vi "Help Center.vi"() -> ()   [LabVIEW 2014]
uses:
  <vilib>/Platform/TimedLoop/XDataNode/timing_clust.ctl
  <vilib>/Platform/TimedLoop/XDataNode/nitl_modes.ctl
  <vilib>/Platform/TimedLoop/XDataNode/wakeup.ctl
  <vilib>/Platform/TimedLoop/XDataNode/XDataNode.xnode
  <vilib>/Platform/TimedLoop/XDataNode/XDNodeRunTimeDep.lvlib
panel:
  in  "Close Button":bool
  in  "Help Tree":string(tree)
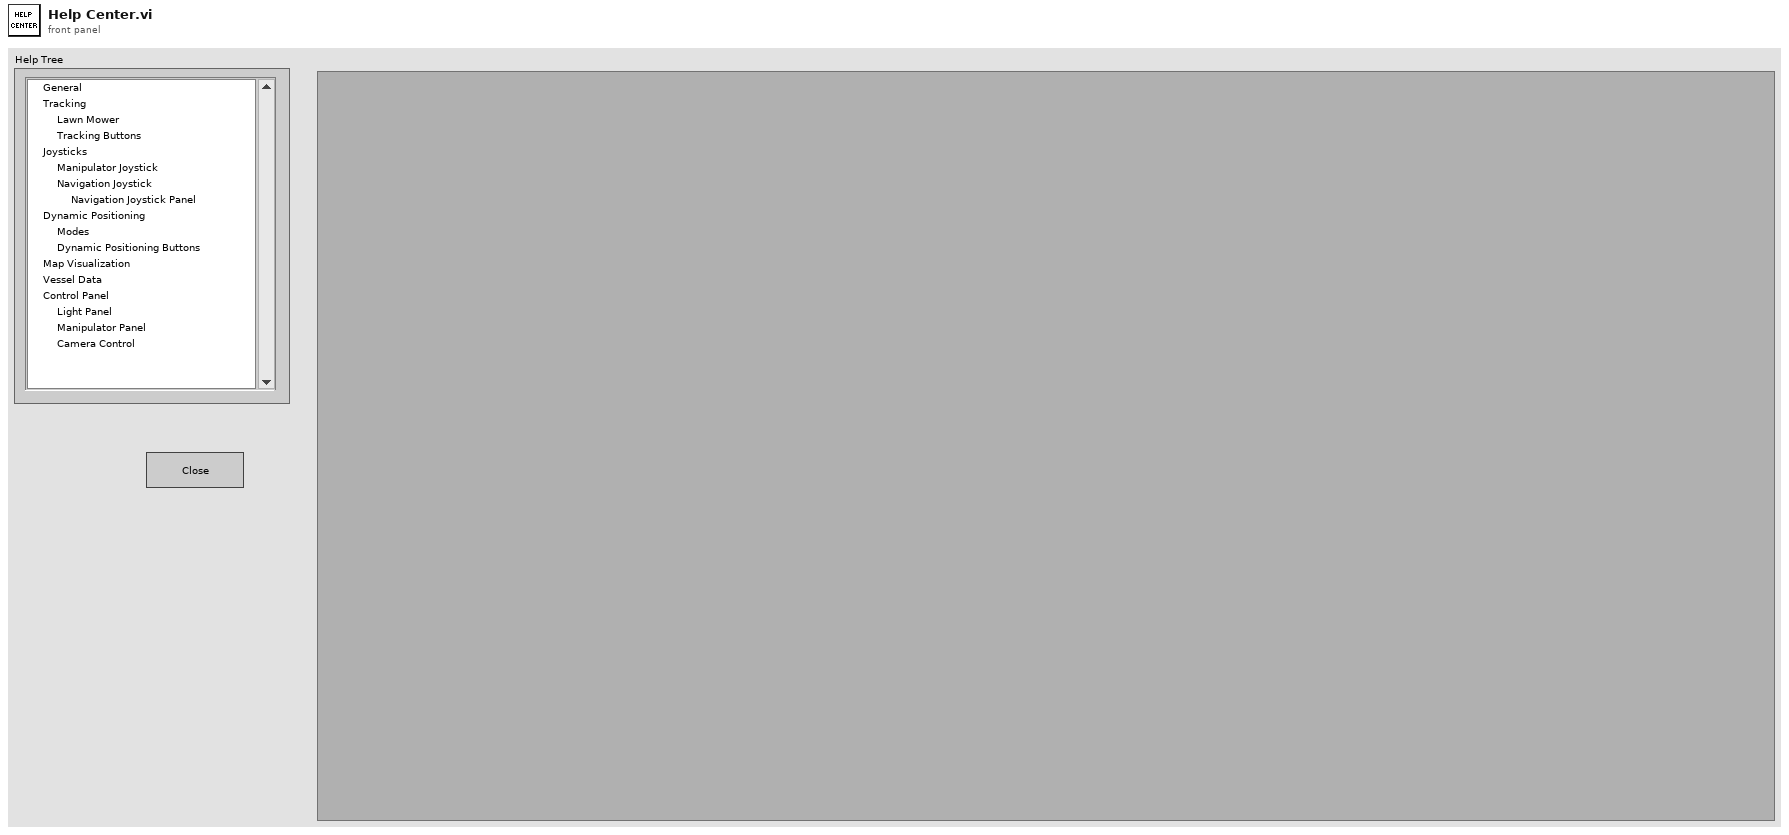
[diagram p1: front panel]
types:
  T1 = typedef "XDNodeRunTimeDep.lvlib/timing_clust.ctl" = cluster{"Expected End [f-1]":u64, "Actual End [f-1]":u64, "Finished Late? [f-1]":bool, "Expected End [i-1]":u64, "Actual End [i-1]":u64, "Finished Late? [i-1]":bool, "Expected Start [i]":u64, "Actual Start [i]":u64, "Expected Start [f]":u64, "Actual Start [f]":u64, "Source Name":string, "Structure Name":string, "Period":i64, "Deadline":i64, "Offset":i64, "Start":i64, "Priority":i32, "Timeout":i32, "Mode":T2, "Wakeup Reason":T3, "Error":errorcluster, "Source Type":string, "Secondary Source Type":string, "Global End Time":u64, "Global Start Time":u64, "Frame Duration":u64, "Iteration Duration":u64, "Assigned CPU":i32, "I/O Scan Engine Mode":u32}
  T2 = typedef "XDNodeRunTimeDep.lvlib/nitl_modes.ctl" = enum32{"No Change", "Process missed periods, maintain original phase", "Discard missed periods, maintain original phase", "Process missed periods, ignore original phase", "Discard missed periods, ignore original phase"}
  T3 = typedef "XDNodeRunTimeDep.lvlib/wakeup.ctl" = enum32{"Normal", "Aborted", "Asynchronous wakeup", "Timing source error", "Timed loop error", "Timeout"}
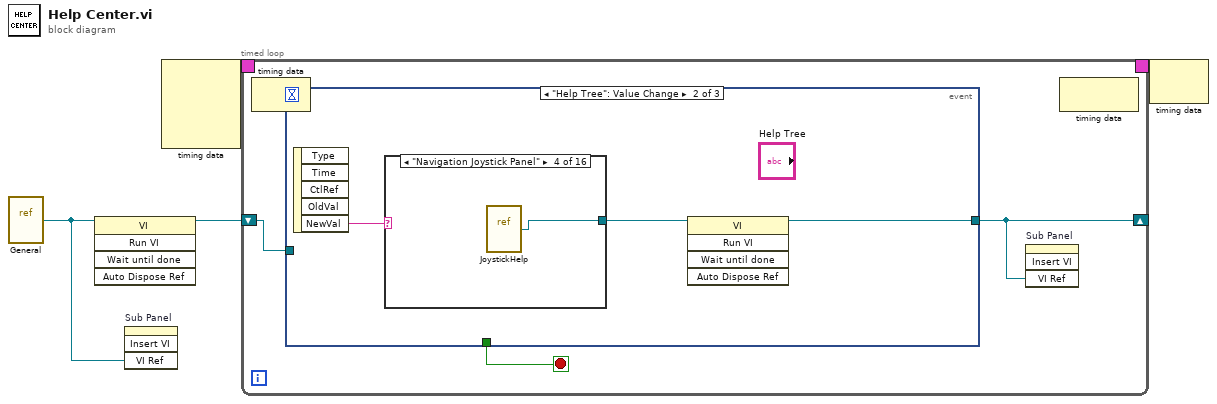
[diagram p0: block diagram]
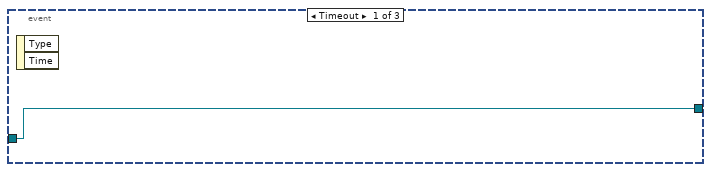
[diagram p2: hidden frame]
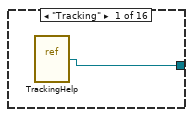
[diagram p3: hidden frame]
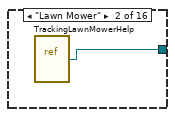
[diagram p4: hidden frame]
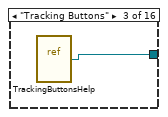
[diagram p5: hidden frame]
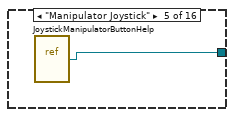
[diagram p6: hidden frame]
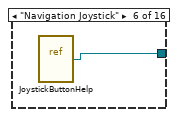
[diagram p7: hidden frame]
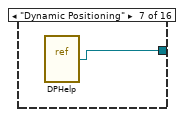
[diagram p8: hidden frame]
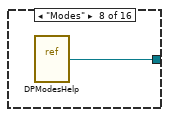
[diagram p9: hidden frame]
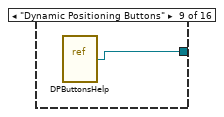
[diagram p10: hidden frame]
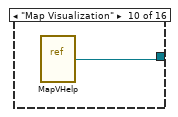
[diagram p11: hidden frame]
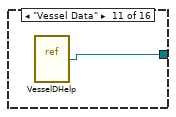
[diagram p12: hidden frame]
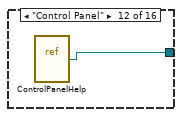
[diagram p13: hidden frame]
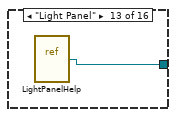
[diagram p14: hidden frame]
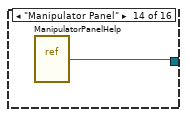
[diagram p15: hidden frame]
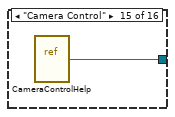
[diagram p16: hidden frame]
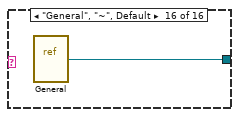
[diagram p17: hidden frame]
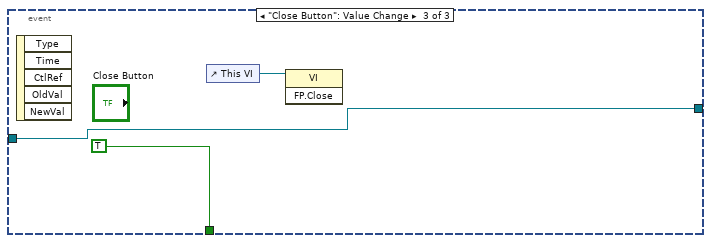
[diagram p18: hidden frame]
diagram:
  n1 = vi-ref "General.vi"() -> (w3:refnum<vi>)
  n2 = invoke class="VI" method="Run VI"(reference=w3) -> (reference out=w4:refnum<vi>)  [unwired: 4 in, 4 out]
  n3 = invoke on="Sub Panel" class="SubPnl" method="Insert VI"("VI Ref"=w3) -> ()  [unwired: 3 in, 4 out]
  n4 = node-c288() -> (w2:T1)  [unwired: 4 in]
  n5 = timed-loop {
    shift-right: [w6] -> _
    shift-left: w4 -> [w5]
    timing: w2 -> [_]
    timing-out: [_] -> w1
    stop <- w7 stop-if-true
    n6 = node-c288() -> ()  [unwired: 1 in, 1 out]
    n7 = event shown="[1] \"Help Tree\": Value Change" {
      selector: _ -> [_ _ _]
      dyn-events: _ -> [_ _ _]
      timeout: _ -> [_ _ _]
      tunnel: [_ _ TRUE] -> w7
      tunnel: [w10 w11 w30] -> w6
      tunnel: w5 -> [w10 _ w30]
      event Timeout {
        n8 = event-data() -> ()  [unwired: 1 in, 2 out]
      }
      event "Help Tree": Value Change {
        n9 = event-data() -> ("NewVal"=w13:string)  [unwired: 1 in, 4 out]
        n10 = case shown="\"Navigation Joystick Panel\"" w13 {
          tunnel: [w14 w15 w16 w17 w18 w19 w20 w21 w22 w23 w24 w25 w26 w27 w28 w29] -> w12
          frame "Tracking" {
            n11 = vi-ref "TrackingHelp.vi"() -> (w14:refnum<vi>)
          }
          frame "Lawn Mower" {
            n12 = vi-ref "TrackingLawnMowerHelp.vi"() -> (w15:refnum<vi>)
          }
          frame "Tracking Buttons" {
            n13 = vi-ref "TrackingButtonsHelp.vi"() -> (w16:refnum<vi>)
          }
          frame "Navigation Joystick Panel" {
            n14 = vi-ref "JoystickHelp.vi"() -> (w17:refnum<vi>)
          }
          frame "Manipulator Joystick" {
            n15 = vi-ref "JoystickManipulatorButtonHelp.vi"() -> (w18:refnum<vi>)
          }
          frame "Navigation Joystick" {
            n16 = vi-ref "JoystickButtonHelp.vi"() -> (w19:refnum<vi>)
          }
          frame "Dynamic Positioning" {
            n17 = vi-ref "DPHelp.vi"() -> (w20:refnum<vi>)
          }
          frame "Modes" {
            n18 = vi-ref "DPModesHelp.vi"() -> (w21:refnum<vi>)
          }
          frame "Dynamic Positioning Buttons" {
            n19 = vi-ref "DPButtonsHelp.vi"() -> (w22:refnum<vi>)
          }
          frame "Map Visualization" {
            n20 = vi-ref "MapVHelp.vi"() -> (w23:refnum<vi>)
          }
          frame "Vessel Data" {
            n21 = vi-ref "VesselDHelp.vi"() -> (w24:refnum<vi>)
          }
          frame "Control Panel" {
            n22 = vi-ref "ControlPanelHelp.vi"() -> (w25:refnum<vi>)
          }
          frame "Light Panel" {
            n23 = vi-ref "LightPanelHelp.vi"() -> (w26:refnum<vi>)
          }
          frame "Manipulator Panel" {
            n24 = vi-ref "ManipulatorPanelHelp.vi"() -> (w27:refnum<vi>)
          }
          frame "Camera Control" {
            n25 = vi-ref "CameraControlHelp.vi"() -> (w28:refnum<vi>)
          }
          frame "General", "~", Default {
            n26 = vi-ref "General.vi"() -> (w29:refnum<vi>)
          }
        }
        n27 = invoke class="VI" method="Run VI"(reference=w12) -> (reference out=w11:refnum<vi>)  [unwired: 4 in, 4 out]
      }
      event "Close Button": Value Change {
        n28 = event-data() -> ()  [unwired: 1 in, 5 out]
        n29 = control-ref of="This VI"() -> (w31:refnum<vi>)
        n30 = invoke class="VI" method="FP.Close"(reference=w31) -> ()  [unwired: 2 in, 3 out]
      }
    }
    n31 = invoke on="Sub Panel" class="SubPanel" method="Insert VI"("VI Ref"=w6) -> ()  [unwired: 3 in, 4 out]
    n32 = node-c288() -> ()  [unwired: 1 in, 1 out]
  }
  n33 = node-c288(w1) -> ()  [unwired: 1 out]
